vi "Read XY unit scale factor.vi"(8 "error in (no error)":errorcluster, 11 "XYCalFactor in":refnum<class "XYCalFactor.lvclass">) -> (0 "error out":errorcluster, 2 "XY unit scale factor":dbl, 3 "XYCalFactor out":refnum<class "XYCalFactor.lvclass">)   [LabVIEW 2013, in "MaterialCharacterization.lvlib" / "XYCalFactor.lvclass"]
uses:
  XYCalFactor.lvclass
  XYCalFactor.lvclass/XYCalFactor.ctl
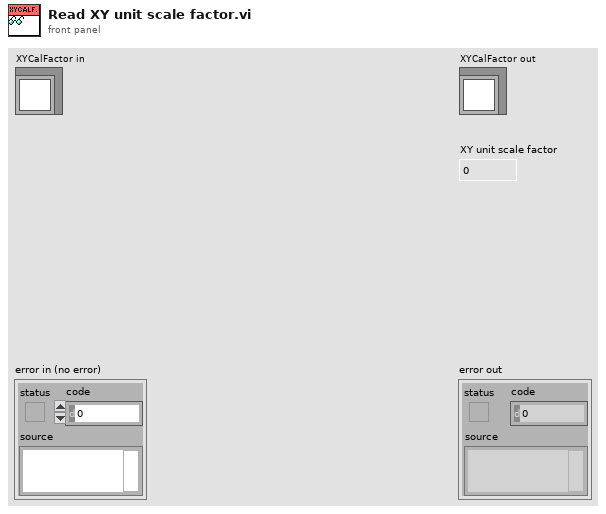
[diagram p1: front panel]
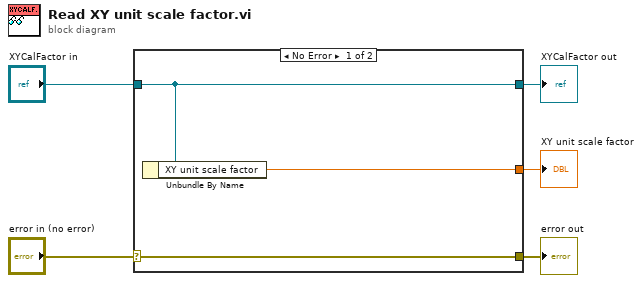
[diagram p0: block diagram]
diagram:
  n1 = case shown="No Error" "error in (no error)" {
    selector: "error in (no error)" -> [w8 w9]
    tunnel: [w8 w9] -> w4
    tunnel: [w7 w10] -> w2
    tunnel: "XYCalFactor in" -> [w7 w10]
    tunnel: [w6 _] -> w1
    frame No Error {
      n2 = Unbundle By Name(w7) -> ("XY unit scale factor"=w6:dbl)
    }
    frame Error {
    }
  }
  "error out" <- w4
  "XYCalFactor out" <- w2
  "XY unit scale factor" <- w1
